vi "Remove Out of Order GPIO Timestamps.vi"(0 "gpio timestamps in":T1[](array[typedef])) -> (4 "gpio timestamps out":T1[](array[typedef]), 6 "out of order timestamps detected":bool)   [LabVIEW 2023, in "GettingStarted_Common_148X_Host.lvlib"]
uses:
  GettingStarted_Common_148X_Host.lvlib
  <instrlib>/FlexRIO/CSI-2/v2/Host/Types/Host GPIO Bank Timestamp.ctl
  <instrlib>/FlexRIO/CSI-2/v2/FPGA/Types/Timestamp ID.ctl
  <instrlib>/FlexRIO/CSI-2/v2/FPGA/Types/GPIO Bank.ctl
  <instrlib>/FlexRIO/CSI-2/v2/Host/NI CSI-2 API Host v2.lvlib
  <instrlib>/FlexRIO/CSI-2/v2/FPGA/NI CSI-2 API FPGA v2.lvlib
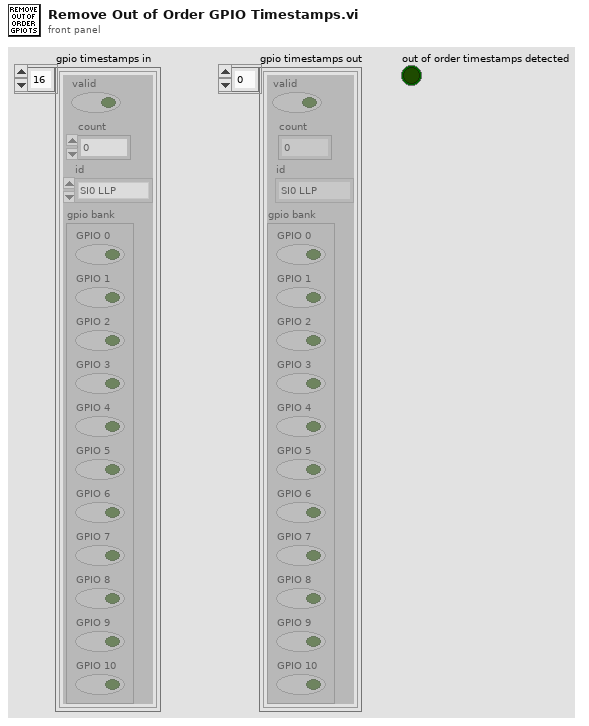
[diagram p1: front panel]
types:
  T1 = typedef "NI CSI-2 API Host v2.lvlib/Host GPIO Bank Timestamp.ctl" = cluster{"valid":bool, "count":u64, "id":T2, "gpio bank":T3}
  T2 = typedef "NI CSI-2 API FPGA v2.lvlib/Timestamp ID.ctl" = enum8{"SI0 LLP", "SI1 LLP", "SI2 LLP", "SI3 LLP", "SI4 LLP", "SI5 LLP", "SI6 LLP", "SI7 LLP", "SO0 LLP", "SO1 LLP", "SO2 LLP", "SO3 LLP", "SO4 LLP", "SO5 LLP", "SO6 LLP", "SO7 LLP", "Ser0 GPIO Bank", "Ser1 GPIO Bank", "Ser2 GPIO Bank", "Ser3 GPIO Bank", "Ser4 GPIO Bank", "Ser5 GPIO Bank", "Ser6 GPIO Bank", "Ser7 GPIO Bank", "Des0 GPIO Bank", "Des1 GPIO Bank", "Des2 GPIO Bank", "Des3 GPIO Bank", "Des4 GPIO Bank", "Des5 GPIO Bank", "Des6 GPIO Bank", "Des7 GPIO Bank", "User0", "User1", "User2", "User3", "User4", "User5", "User6", "User7", "User8", "User9", "User10", "User11", "User12", "User13", "User14", "User15", "User16", "User17", "User18", "User19", "User20", "User21", "User22", "User23", "User24", "User25", "User26", "User27", "User28", "User29", "User30", "User31"}
  T3 = typedef "NI CSI-2 API FPGA v2.lvlib/GPIO Bank.ctl" = cluster{"GPIO 0":bool, "GPIO 1":bool, "GPIO 2":bool, "GPIO 3":bool, "GPIO 4":bool, "GPIO 5":bool, "GPIO 6":bool, "GPIO 7":bool, "GPIO 8":bool, "GPIO 9":bool, "GPIO 10":bool}
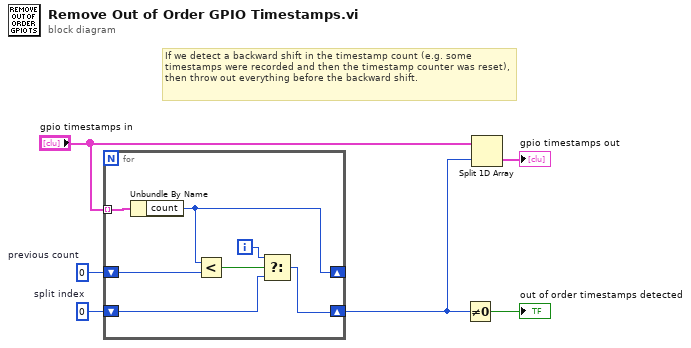
[diagram p0: block diagram]
diagram:
  w3 = 0  # split index
  w4 = u64 0  # previous count
  # "If we detect a backward shift in the timestamp count (e.g. some timestamps were recorded and then the timestamp counter was reset), then throw out everything before the backward shift."
  n1 = for {
    tunnel: "gpio timestamps in" -> [w13] mode=indexing
    shift-right: [w8] -> _
    shift-left: w4 -> [w7]
    shift-right: [w10] -> w1
    shift-left: w3 -> [w11]
    i -> [w12]
    n2 = Unbundle By Name(w13) -> ("count"=w8:u64)
    n3 = Less?(x=w8, y=w7) -> (x < y?=w9:bool)
    n4 = Select(t=w12, s=w9, f=w11) -> (s? t:f=w10:i32)
  }
  n5 = Not Equal To 0?(x=w1) -> (x != 0?=→"out of order timestamps detected":bool)
  n6 = Split 1D Array(array="gpio timestamps in", index=w1) -> (second subarray=→"gpio timestamps out":T1[])  [unwired: 1 out]
